vi "PeakAt.vi"(10 "Index":u32, 11 "POTTypedCircularBuffer in":refnum<class "ErrorLogBuffer.lvclass">) -> (2 "element":T1, 3 "POTTypedCircularBuffer out":refnum<class "ErrorLogBuffer.lvclass">)   [LabVIEW 2024, in "ErrorLogBuffer.lvclass"]
uses:
  ErrorLogBuffer.lvclass
  RQMHCore/ErrorReporting/Record/LogRecord.lvclass
  ErrorLogBuffer.lvclass/ErrorLogBuffer.ctl
  Type.ctl
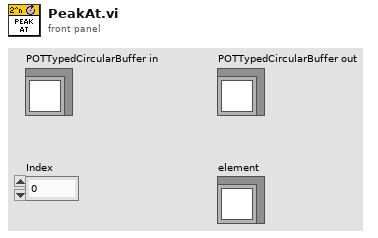
[diagram p1: front panel]
types:
  T1 = typedef "ErrorLogBuffer.lvclass/Type.ctl" = refnum<class "LogRecord.lvclass">
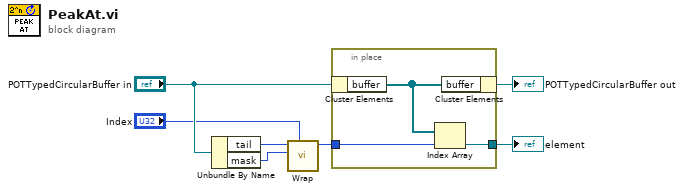
[diagram p0: block diagram]
diagram:
  n1 = Unbundle By Name("POTTypedCircularBuffer in") -> ("tail"=w4:i32, "mask"=w3:i32)
  n2 = call "Wrap.vi"("increment amount (1)"="Index", "mask"=w3, "index"=w4) -> ("wrapped"=w1:i32)  [unwired: 8 in]
  n3 = in-place {
    in-place-border: [w9] -> w6
    in-place-border: w1 -> [w8]
    n4 = in-place-cluster #1("POTTypedCircularBuffer in") -> ("buffer"=w10:T1[])
    n5 = Index Array(array=w10, index=w8) -> (element=w9:T1)
    n6 = in-place-cluster #1("buffer"=w10) -> (→"POTTypedCircularBuffer out":refnum<class "ErrorLogBuffer.lvclass">)
  }
  "element" <- w6
